vi "8164B Read Power.vi"(8 "error in":errorcluster, 11 "KeySight 8164B control in":T1) -> (0 "error out":errorcluster, 2 "Power":dbl format="%#_6p", 3 "KeySight 8164B control out":T1)   [LabVIEW 2018, in "KeySight 8164B LAN InstrLib.lvlib"]
uses:
  KeySight 8164B LAN InstrLib.lvlib
  typedefs/KeySight 8164B control.ctl
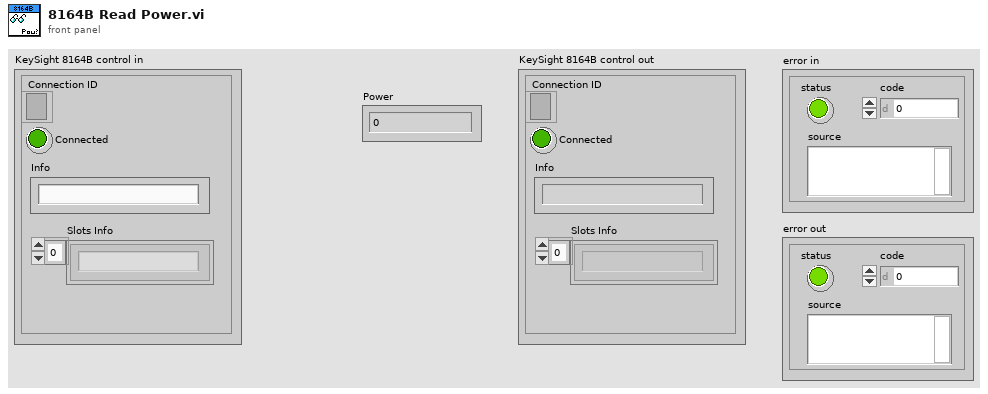
[diagram p1: front panel]
types:
  T1 = typedef "KeySight 8164B LAN InstrLib.lvlib/KeySight 8164B control.ctl" = cluster{"Connection ID":refnum<k5>, "Connected":bool, "Info":string, "Slots Info":string[]}
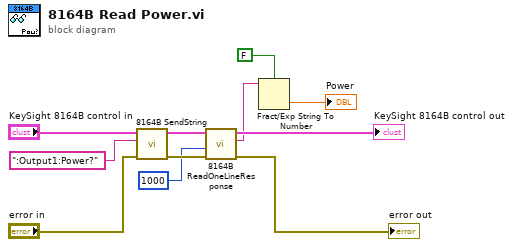
[diagram p0: block diagram]
diagram:
  n1 = call "8164B SendString.vi"("error in"="error in", "CMD"=":Output1:Power?", "KeySight 8164B control in"="KeySight 8164B control in") -> ("error out"=w6:errorcluster, "KeySight 8164B control out"=w8:T1)  [unwired: 7 in]
  n2 = call "8164B ReadOneLineResponse.vi"("error in"=w6, "timeout ms"=1000 ("timeout ms (25000)"), "KeySight 8164B control in"=w8) -> ("error out"=→"error out":errorcluster, "OneLineResponse"=w2:string, "KeySight 8164B control out"=→"KeySight 8164B control out":T1)  [unwired: 6 in]
  n3 = Fract/Exp String To Number(use system decimal point (T)=FALSE, string=w2) -> (number=→"Power":dbl)  [unwired: 2 in, 1 out]
